vi "C844_SetPara_modified_Amit.vi"(3 "Error in":errorcluster, 5 "P-term   i-term   d-term   Accel.":u32[][](array[numeric])=[[250, 12, 200, 65000, 850000], [250, 12, 200, 50000, 850000], [250, 12, 200, 50000, 850000], [250, 12, 200, 50000, 850000]]) -> (0 "Error out":errorcluster)   [LabVIEW 2009]
doc: "Sets p-i-d-parameters, velocities and accelerations for all 4 axes"
panel:
  out "Control string":string
  # "C-844 Set Parameters"
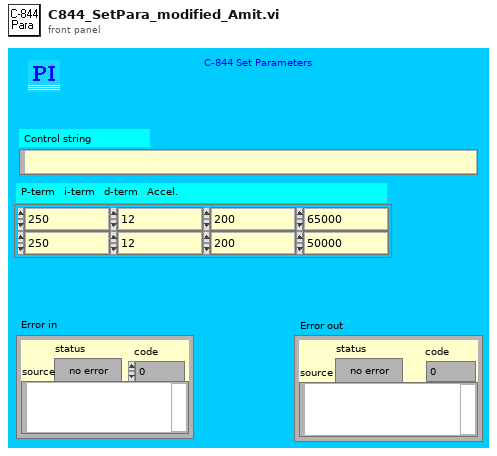
[diagram p1: front panel]
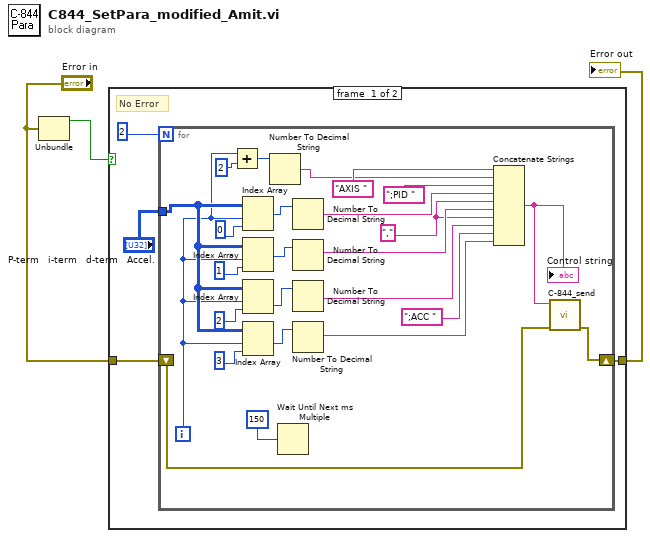
[diagram p0: block diagram]
diagram:
  n1 = Unbundle("Error in") -> ("status"=w3:bool)  [unwired: 2 out]
  n2 = case shown="False" w3 {
    tunnel: "Error in" -> [w5 w33]
    tunnel: [w4 w33] -> w2
    frame #0 {
      # "No Error"
      n3 = for {
        N: u8 2 -> [_]
        tunnel: "P-term   i-term   d-term   Accel." -> [w17]
        shift-right: [w12] -> w4
        shift-left: w5 -> [w11]
        i -> [w10]
        w21 = ","
        n4 = Add(x=w10, y=2) -> (x+y=w9:i32)
        n5 = Index Array(array=w17, index (row)=w10, index (col)=0) -> (element=w26:u32)
        n6 = Index Array(array=w17, index (row)=w10, index (col)=1) -> (element=w25:u32)
        n7 = Index Array(array=w17, index (row)=w10, index (col)=2) -> (element=w24:u32)
        n8 = Index Array(array=w17, index (row)=w10, index (col)=3) -> (element=w18:u32)
        n9 = Number To Decimal String(number=w9) -> (decimal integer string=w28:string)  [unwired: 1 in]
        n10 = Wait Until Next ms Multiple(millisecond multiple=150) -> ()  [unwired: 1 out]
        n11 = Number To Decimal String(number=w26) -> (decimal integer string=w23:string)  [unwired: 1 in]
        n12 = Number To Decimal String(number=w25) -> (decimal integer string=w22:string)  [unwired: 1 in]
        n13 = Number To Decimal String(number=w24) -> (decimal integer string=w20:string)  [unwired: 1 in]
        n14 = Number To Decimal String(number=w18) -> (decimal integer string=w15:string)  [unwired: 1 in]
        n15 = Concatenate Strings("AXIS ", w28, ";PID ", w23, w21, w22, w21, w20, ";ACC ", w15) -> (w13:string)
        "Control string" <- w13
        n16 = call "C-844_send.vi"("error in (no error)"=w11, "Command"=w13) -> ("error out"=w12:errorcluster)  [unwired: 7 in, 2 out]
      }
    }
    frame #1 {
      # "Error prior execution"
      # "Error"
    }
  }
  "Error out" <- w2
